vi "getBitAsBoolean.vi"(10 "n":i32=-1, 11 "input":u8 format="%08b") -> (3 "bit":bool)   [LabVIEW 2013, in "bitwiseOps.lvlib"]
uses:
  bitwiseOps.lvlib
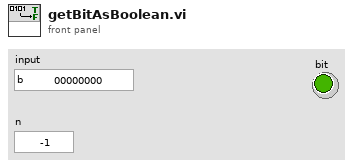
[diagram p1: front panel]
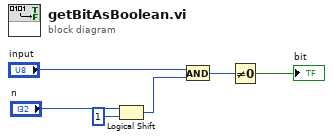
[diagram p0: block diagram]
diagram:
  n1 = Logical Shift(y="n", x=u8 1) -> (x << y=w5:u8)
  n2 = And(x="input", y=w5) -> (x .and. y?=w3:u8)
  n3 = Not Equal To 0?(x=w3) -> (x != 0?=→"bit":bool)
